vi "UDP Factory.vi"(8 "error in (no error)":errorcluster, 10 "settings":T1) -> (0 "error out":errorcluster, 3 "protocol out":refnum<class "Protocol Parent.lvclass">)   [LabVIEW 2019, in "Instrument Addon Scripting API.lvlib"]
doc: "Instantiates a new UPD Protocol object using the provided UDP settings."
uses:
  Instrument Addon Scripting API.lvlib
  Includes/Protocols.lvlibp/UDP/UDP Settings.ctl
  Includes/Protocols.lvlibp/Protocol Parent/Protocol Parent.lvclass
  Includes/Protocols.lvlibp/UDP/UDP.lvclass
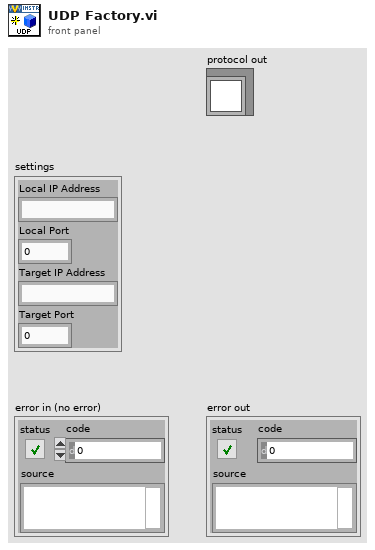
[diagram p1: front panel]
types:
  T1 = typedef "Protocols.lvlibp/UDP.lvclass/UDP Settings.ctl" = cluster{"Local IP Address":string, "Local Port":u16, "Target IP Address":string, "Target Port":u16}
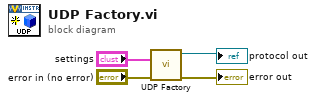
[diagram p0: block diagram]
diagram:
  n1 = call "UDP Factory.vi"("error in (no error)"="error in (no error)", "UDP settings"="settings") -> ("error out"=→"error out":errorcluster, "protocol out"=→"protocol out":refnum<class "Protocol Parent.lvclass">)  [unwired: 8 in]
